vi "ADCP_UI_Continuous_Transmitter_Core.vi"(8 "error in (no error)":errorcluster, 11 "Initialize ?":bool) -> (0 "error out":errorcluster, 3 "Packets":cluster{"Packet Bytes":u8[]}[](array[cluster]))   [LabVIEW 2017]
uses:
  Controls/Data Packets/Data_Packet_FGV_Commands.ctl
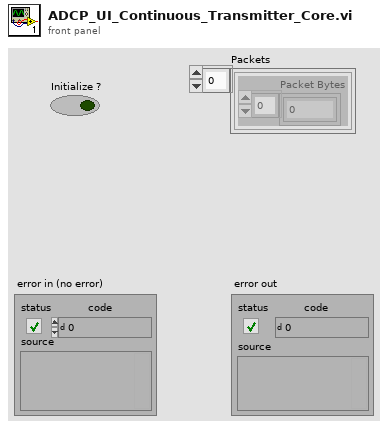
[diagram p1: front panel]
types:
  T1 = typedef "Data_Packet_FGV_Commands.ctl" = enum16{"Update all parameters from data packets", "Update Packet", "Load", "Read Packet Parameters", "Write Packet Parameters", "Read Packet Parameter", "Write Packet Parameter", "Read Data Packets", "Read Data Packet", "Read Data Packet by Parameter Name", "Get Parameter Node and Frame ID", "Read Data Packet from Node ID and Frame ID"}
  T2 = typedef "Data_Packet.ctl" = cluster{"Packet":T3, "Parameters":T7[], "Last Received Time (ms)":u64, "Receive count":i32, "Transmit count":i32, "Transmit interval (ms)":u32, "Last Transmitted Time (ms)":u64, "Receive interval (ms)":u32, "Transmit_Mode":T9, "Transmit Enable":bool, "Cyclic Transmit interval (ms)":u32}
  T3 = typedef "Packet.ctl" = cluster{"Raw Bytes":u8[], "Checksum":bool, "Direction":T4, "Processed Bytes":u8[], "Node ID":u8, "Packet type":T5, "Frame Data":u32, "Priority":T6, "Frame ID":u8}
  T4 = typedef "Packet_Direction.ctl" = enum16{"Transmit", "Receive", "Bidirectional"}
  T5 = typedef "Packet_Type.ctl" = enum16{"Data", "Connection Management", "Remote Request", "Error/Status"}
  T6 = typedef "Packet_Priority.ctl" = enum16{"LOW", "HIGH"}
  T7 = typedef "Parameter.ctl" = cluster{"Parameter name":string, "Node name":string, "Node ID":u8, "Frame name":string, "Frame ID":u8, "Data type":T8, "Start Bit":i32, "Bit Length":i32, "Factor":dbl, "Offset":dbl, "Minimum":dbl, "Maximum":dbl, "Descriptor":string, "Enum values":string[], "Value":string}
  T8 = typedef "Parameter_Data_Type.ctl" = enum16{"BOOL", "UNSIGNED", "SIGNED", "FLOAT32", "ENUM"}
  T9 = typedef "Data_Packet_Transmit_Mode.ctl" = enum16{"Disabled", "Single", "Cyclic"}
  T10 = typedef "ADCP_UI_Data_Packet_Transmitter_Parameters.ctl" = cluster{"Node ID":u32, "Frame ID":u32, "Count":u32, "Last transmitted time (ms)":u32, "Time interval (ms)":u32}
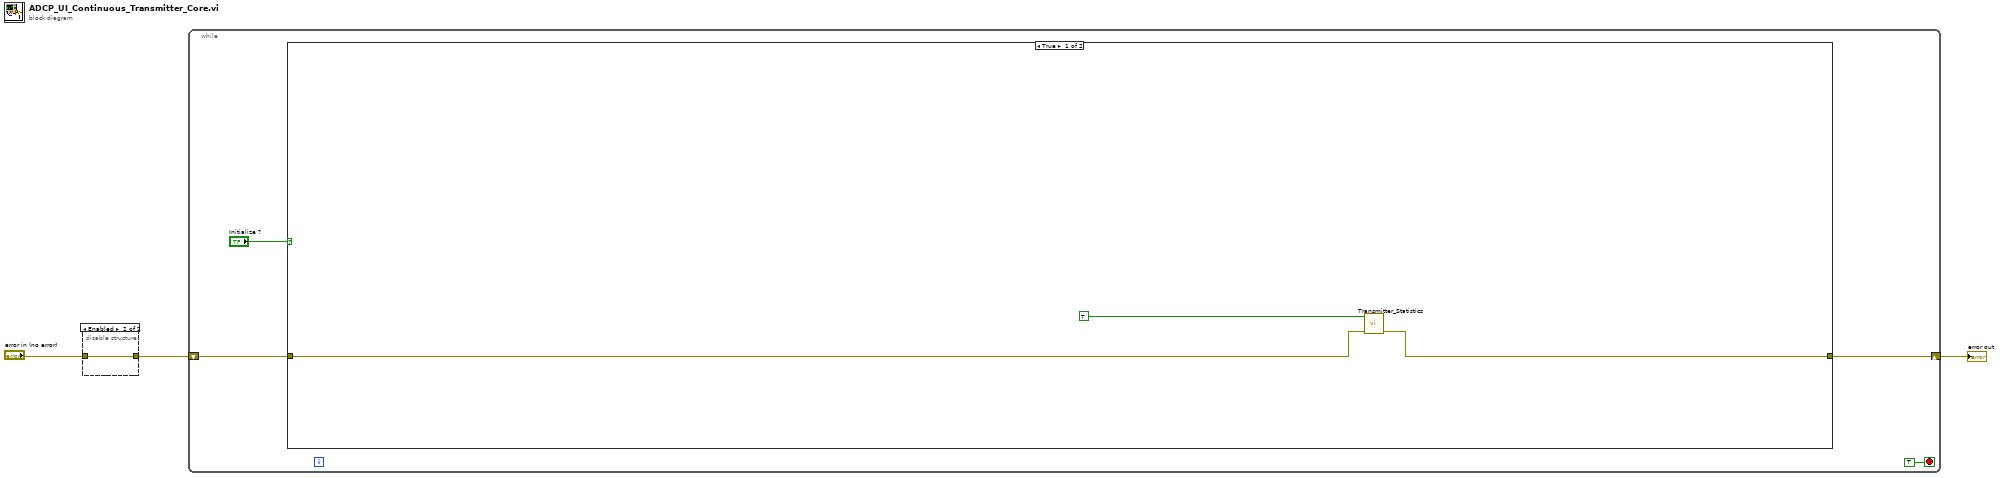
[diagram p0: block diagram]
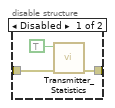
[diagram p2: hidden frame]
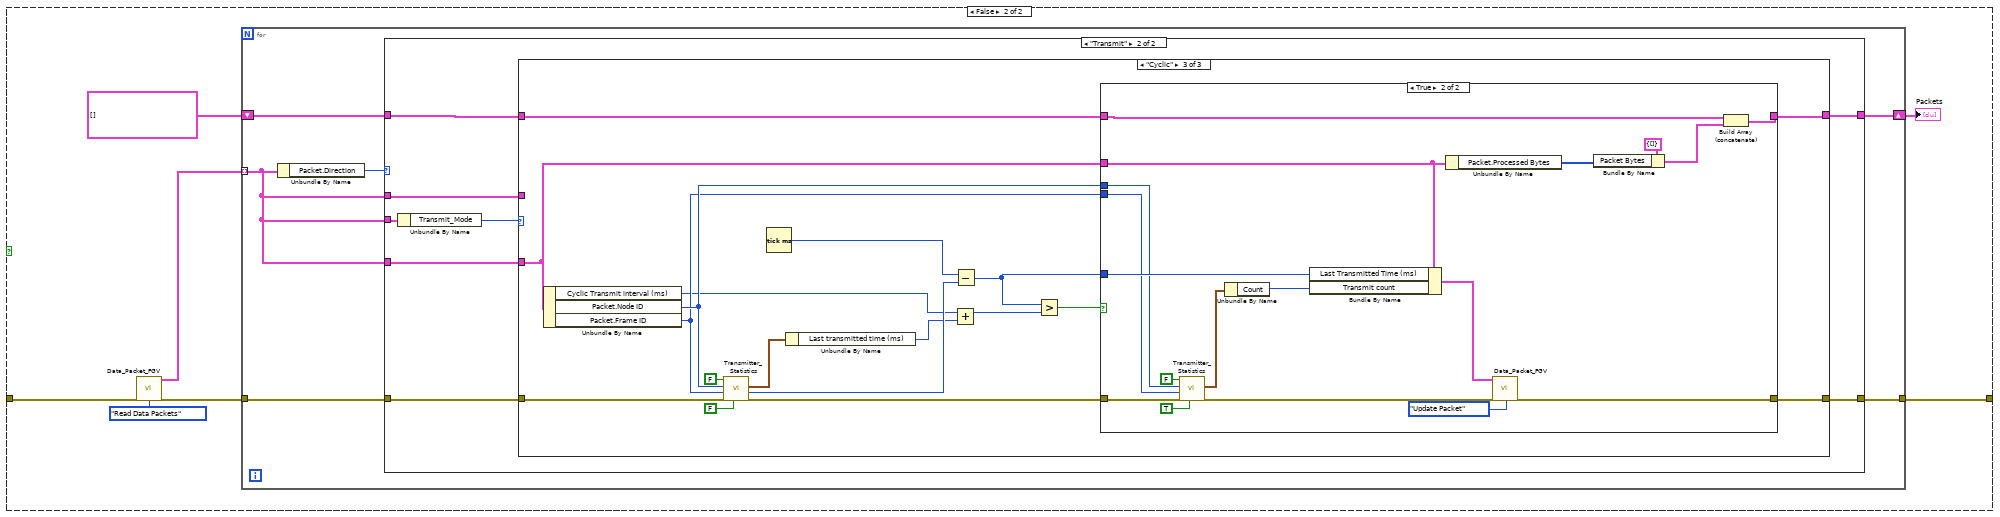
[diagram p3: hidden frame]
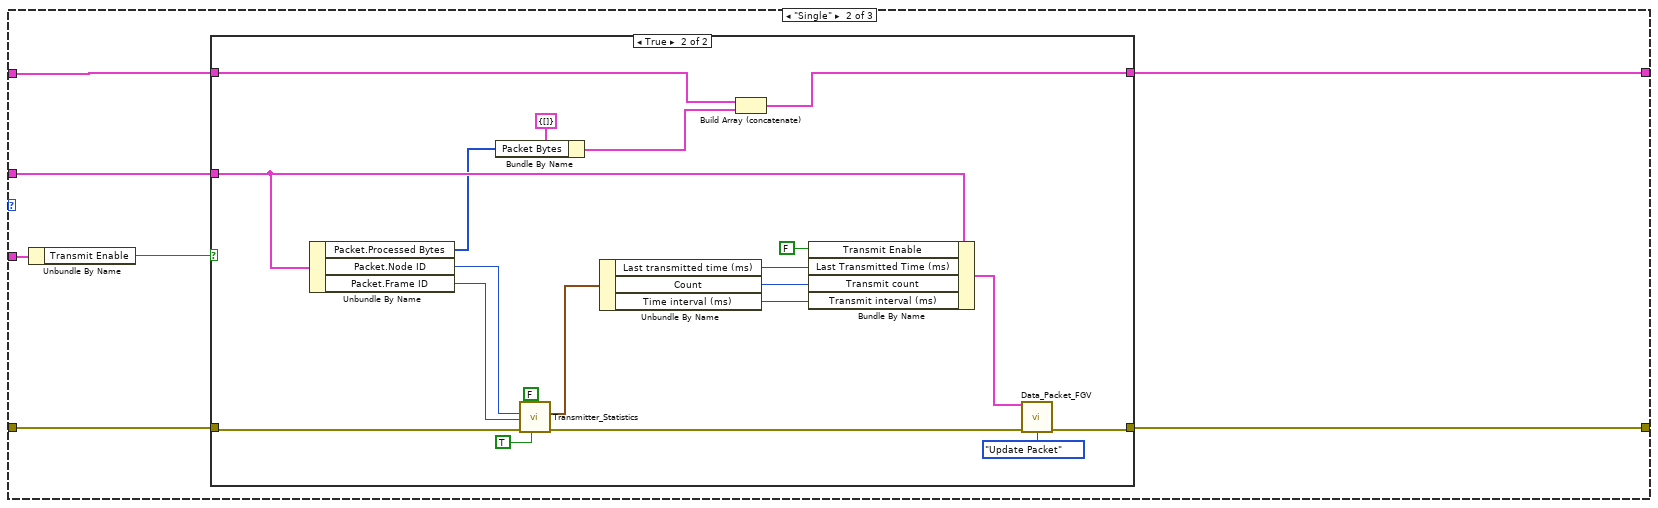
[diagram p6: hidden frame]
diagram:
  n1 = disable-structure shown="Enabled" {
    disable-tunnel: "error in (no error)" -> [w6 w7]
    disable-tunnel: [w5 w7] -> w1
    frame Disabled {
      n2 = call "Transmitter_Statistics.vi"("error in (no error)"=w6, "Initialize ?"=TRUE) -> ("error out"=w5:errorcluster)  [unwired: 6 in, 3 out]
    }
    frame Enabled {
    }
  }
  n3 = while {
    shift-right: [w9] -> w3
    shift-left: w1 -> [w11]
    stop <- TRUE stop-if-true
    n4 = case shown="True" "Initialize ?" {
      tunnel: w11 -> [w14 w21]
      tunnel: [w13 w16] -> w9
      frame True {
        n5 = call "Transmitter_Statistics.vi"("error in (no error)"=w14, "Initialize ?"=TRUE) -> ("error out"=w13:errorcluster)  [unwired: 6 in, 3 out]
      }
      frame False {
        n6 = call "Data_Packet_FGV.vi"("error in (no error)"=w21, "Commands"=Data_Packet_FGV_Commands."Read Data Packets") -> ("Data Packets Out"=w18:T2[], "error out"=w19:errorcluster)  [unwired: 8 in, 4 out]
        n7 = for {
          tunnel: w19 -> [w26]
          tunnel: w18 -> [w24] mode=indexing
          tunnel: [w25] -> w16
          shift-right: [w22] -> w15
          shift-left: cluster{"Packet Bytes":u8[]}[] [] -> [w23]
          n8 = Unbundle By Name(w24) -> ("Packet.Direction"=w27:T4)
          n9 = case shown="\"Transmit\"" w27 {
            tunnel: w26 -> [w29 w37]
            tunnel: w24 -> [_ w36]
            tunnel: [w29 w33] -> w25
            tunnel: w24 -> [_ w34]
            tunnel: w24 -> [_ w32]
            tunnel: w23 -> [w28 w31]
            tunnel: [w28 w30] -> w22
            frame Default {
            }
            frame "Transmit" {
              n10 = Unbundle By Name(w36) -> ("Transmit_Mode"=w35:T9)
              n11 = case shown="\"Cyclic\"" w35 {
                tunnel: w37 -> [w38 w46 w86]
                tunnel: w34 -> [_ w41 _]
                tunnel: [w38 w45 w78] -> w33
                tunnel: w32 -> [_ w44 w75]
                tunnel: w31 -> [w39 w42 w77]
                tunnel: [w39 w40 w76] -> w30
                frame "Disabled", Default {
                }
                frame "Single" {
                  n12 = Unbundle By Name(w44) -> ("Transmit Enable"=w43:bool)
                  n13 = case shown="True" w43 {
                    tunnel: w46 -> [w47 w63]
                    tunnel: [w47 w67] -> w45
                    tunnel: w42 -> [w48 w53]
                    tunnel: w41 -> [_ w65]
                    tunnel: [w48 w52] -> w40
                    frame False {
                    }
                    frame True {
                      n14 = Unbundle By Name(w65) -> ("Packet.Processed Bytes"=w64:u8[], "Packet.Node ID"=w61:u8, "Packet.Frame ID"=w60:u8)
                      n15 = Bundle By Name(cluster=cluster{"Packet Bytes":u8[]} {"Packet Bytes"=[]} ("Transmit Packet"), "Packet Bytes"=w64) -> (w50:cluster{"Packet Bytes":u8[]})
                      n16 = call "Transmitter_Statistics.vi"("Write ?"=TRUE, "error in (no error)"=w63, "Frame ID"=w60, "Node ID"=w61, "Initialize ?"=FALSE) -> ("error out"=w62:errorcluster, "Output"=w57:T10)  [unwired: 3 in, 2 out]
                      n17 = Unbundle By Name(w57) -> ("Last transmitted time (ms)"=w56:u32, "Count"=w55:u32, "Time interval (ms)"=w51:u32)
                      n18 = Build Array (concatenate)(w53, w50) -> (w52:cluster{"Packet Bytes":u8[]}[])
                      n19 = Bundle By Name(cluster=w65, "Transmit Enable"=FALSE, "Last Transmitted Time (ms)"=w56, "Transmit count"=w55, "Transmit interval (ms)"=w51) -> (w49:T2)
                      n20 = call "Data_Packet_FGV.vi"("Data_Packet In"=w49, "error in (no error)"=w62, "Commands"=Data_Packet_FGV_Commands."Update Packet") -> ("error out"=w67:errorcluster)  [unwired: 7 in, 5 out]
                    }
                  }
                }
                frame "Cyclic" {
                  n21 = Unbundle By Name(w75) -> ("Cyclic Transmit interval (ms)"=w70:u32, "Packet.Node ID"=w73:u8, "Packet.Frame ID"=w72:u8)
                  n22 = call "Transmitter_Statistics.vi"("Write ?"=FALSE, "error in (no error)"=w86, "Frame ID"=w72, "Node ID"=w73, "Initialize ?"=FALSE) -> ("error out"=w79:errorcluster, "Start Time (ms)"=w82:u32, "Output"=w83:T10)  [unwired: 3 in, 1 out]
                  n23 = Tick Count (ms)() -> (millisecond timer value=w81:u32)
                  n24 = Unbundle By Name(w83) -> ("Last transmitted time (ms)"=w71:u32)
                  n25 = Add(x=w70, y=w71) -> (x+y=w69:u32)
                  n26 = Subtract(x=w81, y=w82) -> (x-y=w74:u32)
                  n27 = Greater?(x=w74, y=w69) -> (0:w80:bool)
                  n28 = case shown="True" w80 {
                    tunnel: w79 -> [w88 w105]
                    tunnel: [w88 w90] -> w78
                    tunnel: w77 -> [w87 w93]
                    tunnel: [w87 w91] -> w76
                    tunnel: w75 -> [_ w95]
                    tunnel: w74 -> [_ w106]
                    tunnel: w73 -> [_ w101]
                    tunnel: w72 -> [_ w100]
                    frame False {
                    }
                    frame True {
                      n29 = call "Transmitter_Statistics.vi"("Write ?"=TRUE, "error in (no error)"=w105, "Frame ID"=w100, "Node ID"=w101, "Initialize ?"=FALSE) -> ("error out"=w104:errorcluster, "Output"=w99:T10)  [unwired: 3 in, 2 out]
                      n30 = Unbundle By Name(w99) -> ("Count"=w98:u32)
                      n31 = Bundle By Name(cluster=w95, "Last Transmitted Time (ms)"=w106, "Transmit count"=w98) -> (w97:T2)
                      n32 = Unbundle By Name(w95) -> ("Packet.Processed Bytes"=w94:u8[])
                      n33 = call "Data_Packet_FGV.vi"("Data_Packet In"=w97, "error in (no error)"=w104, "Commands"=Data_Packet_FGV_Commands."Update Packet") -> ("error out"=w90:errorcluster)  [unwired: 7 in, 5 out]
                      n34 = Bundle By Name(cluster=cluster{"Packet Bytes":u8[]} {"Packet Bytes"=[]} ("Transmit Packet"), "Packet Bytes"=w94) -> (w89:cluster{"Packet Bytes":u8[]})
                      n35 = Build Array (concatenate)(w93, w89) -> (w91:cluster{"Packet Bytes":u8[]}[])
                    }
                  }
                }
              }
            }
          }
        }
        "Packets" <- w15
      }
    }
  }
  "error out" <- w3
